vi "Close.vi"(8 "error in":errorcluster, 11 "gRPC XNET Read Raw CAN Frame Strategy in":refnum<class "gRPC XNET Read Raw CAN Frame Strategy.lvclass">) -> (0 "error out":errorcluster, 3 "gRPC XNET Read Raw CAN Frame Strategy out":refnum<class "gRPC XNET Read Raw CAN Frame Strategy.lvclass">)   [LabVIEW 2024, in "gRPC XNET Read Raw CAN Frame Strategy.lvclass"]
uses:
  gRPC XNET Read Raw CAN Frame Strategy.lvclass
  gRPC XNET Read Raw CAN Frame Strategy.lvclass/gRPC XNET Read Raw CAN Frame Strategy.ctl
  grpc-xnet/grpc-xnet_client/grpc-xnet_client.lvlib
  grpc-xnet/grpc-xnet_client/RPC Messages/nidevice_grpc_Session.ctl
  grpc-xnet/grpc-xnet_client/RPC Messages/nixnet_grpc_ClearRequest.ctl
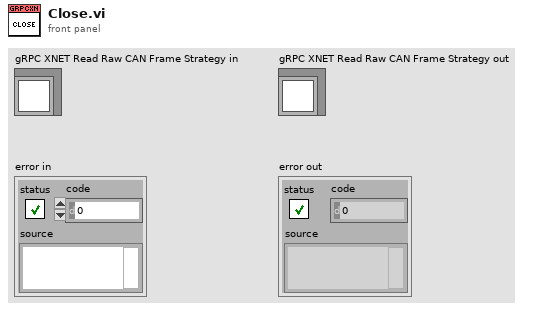
[diagram p1: front panel]
types:
  T1 = typedef "grpc-xnet_client.lvlib/nixnet_grpc_ClearRequest.ctl" = cluster{"session":T2}
  T2 = typedef "grpc-xnet_client.lvlib/nidevice_grpc_Session.ctl" = cluster{"name":string}
  T3 = typedef "grpc-lvsupport-release.lvlib/grpcId.ctl" = u64
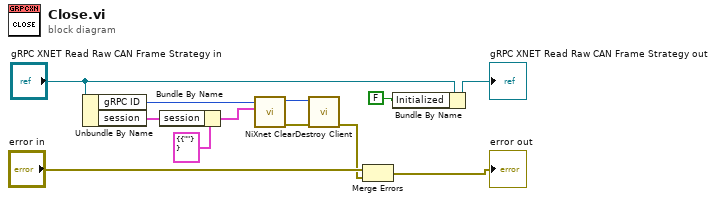
[diagram p0: block diagram]
diagram:
  n1 = Unbundle By Name("gRPC XNET Read Raw CAN Frame Strategy in") -> ("gRPC ID"=w10:T3, "session"=w7:T2)
  n2 = Bundle By Name(cluster=T1 {"session"={"name"=""}} ("Request Data"), "session"=w7) -> (w6:T1)
  n3 = call "NiXnet Clear.vi"("Request Data"=w6, "gRPC ID"=w10) -> ("error out"=w3:errorcluster, "gRPC ID out"=w4:T3)  [unwired: 7 in, 1 out]
  n4 = call "Destroy Client.vi"("error in"=w3, "gRPC ID"=w4) -> ("error out"=w5:errorcluster)  [unwired: 9 in]
  n5 = Merge Errors("error in", w5) -> (→"error out":errorcluster)
  n6 = Bundle By Name(cluster="gRPC XNET Read Raw CAN Frame Strategy in", "Initialized"=FALSE) -> (→"gRPC XNET Read Raw CAN Frame Strategy out":refnum<class "gRPC XNET Read Raw CAN Frame Strategy.lvclass">)
